vi "fg_temp_dir_config.vi"(8 "error in (no error)":errorcluster) -> (0 "error out":errorcluster, 3 "temp_dir_config":T1)   [LabVIEW 2015, in "lv-post-installer.lvlib"]
uses:
  lv-post-installer.lvlib
  public/_controls/temp_dir_config.ctl
  <vilib>/Utility/sysdir.llb/System Directory Type.ctl
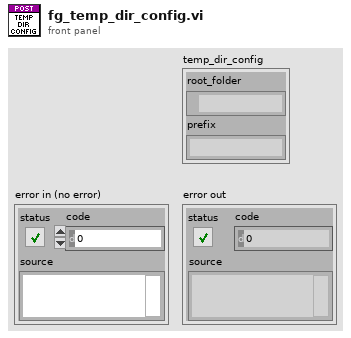
[diagram p1: front panel]
types:
  T1 = typedef "lv-post-installer.lvlib/temp_dir_config.ctl" = cluster{"root_folder":path, "prefix":string}
  T2 = typedef "System Directory Type.ctl" = i32
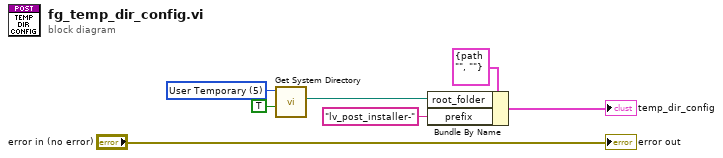
[diagram p0: block diagram]
diagram:
  w3 = T2 5 items=["User Home"=0, "User Desktop"=1, "User Documents"=2, "User Application Data"=3, "User Preferences"=4, "User Temporary"=5, "Public Documents"=6, "Public Application Data"=7, "Public Preferences"=8, "Public Cache"=13, "System Core Libraries"=9, "System Installed Libraries"=10, "Application Files"=11, "Boot Volume Root"=12] ("system directory type")
  n1 = call <vilib>:"Get System Directory.vi"("create directory if not found? (F)"=TRUE, "system directory type"=w3) -> ("system directory"=w4:path)  [unwired: 9 in]
  n2 = Bundle By Name(cluster=T1 {"root_folder"=path "", "prefix"=""} ("temp_dir_config in"), "root_folder"=w4, "prefix"="lv_post_installer-") -> (→"temp_dir_config":T1)
  "error out" <- "error in (no error)"
